vi "Insert_Event_Log(Auto_Event)vi.vi"(10 "[Log] 紀錄Auto流程":T1, 11 "DBlink":string="Driver={ODBC Driver 17 for SQL Server};Server=localhost\\SQLEXPRESS;Database=ZDX905;UID=labview;PWD=Dsa@54137926") -> (0 "error out":errorcluster, 3 "DBlink out":string)   [LabVIEW 2019]
uses:
  <vilib>/addons/database/Connection.llb/DB Tools Open Connec (String).vi
  <vilib>/addons/database/NI_Database_API.lvlib
panel:
  in  "error in (no error)":errorcluster
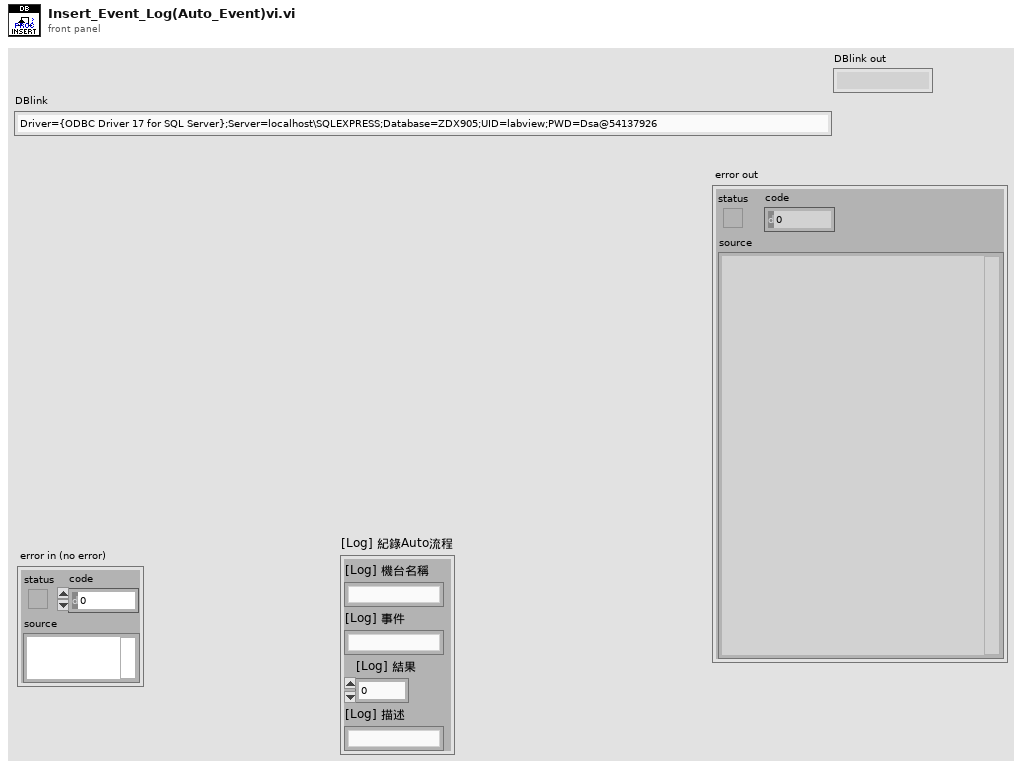
[diagram p1: front panel]
types:
  T1 = cluster{"[Log] 機台名稱":string, "[Log] 事件":string, "[Log] 結果":u16, "[Log] 描述":string}
  T2 = typedef "NI_Database_API.lvlib/Conn ObjectReference.ctl" = refnum<k1>
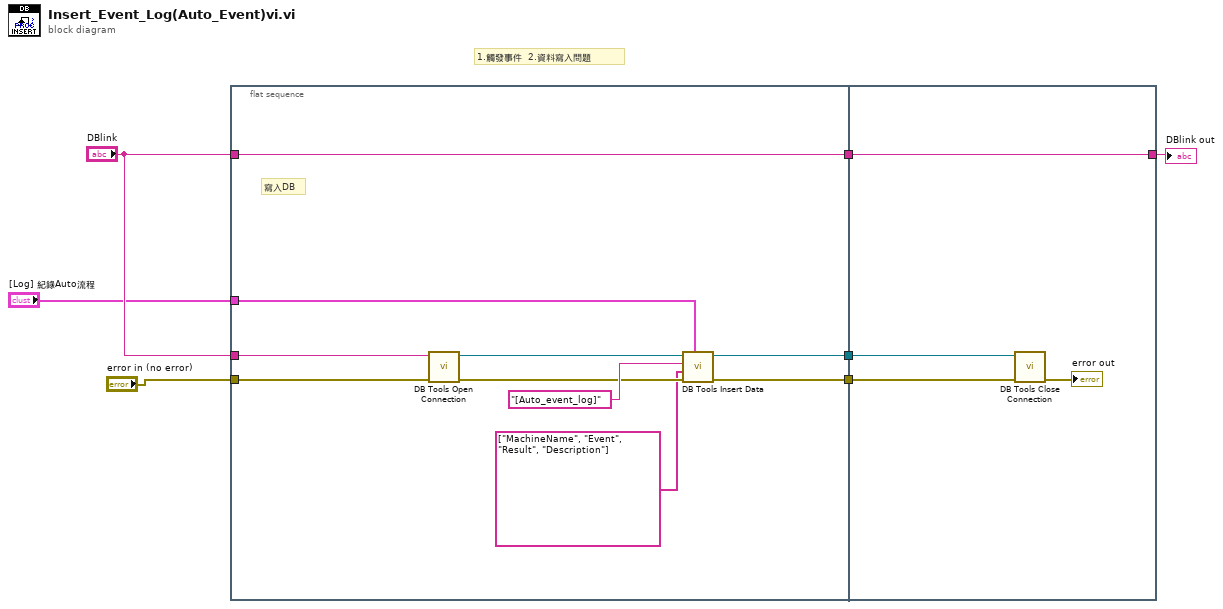
[diagram p0: block diagram]
diagram:
  # "1.觸發事件  2.資料寫入問題"
  n1 = flat-sequence {
    tunnel: [w16] -> w7
    tunnel: [w17] -> w6
    tunnel: "error in (no error)" -> [w11]
    tunnel: "DBlink" -> [w10]
    tunnel: "DBlink" -> [w9]
    tunnel: [w9] -> w3
    tunnel: "[Log] 紀錄Auto流程" -> [w8]
    tunnel: w7 -> [w19]
    tunnel: w6 -> [w20]
    tunnel: w3 -> [w18]
    tunnel: [w18] -> w2
    frame #0 {
      # "寫入DB"
      n2 = call-poly <vilib>:"DB Tools Open Connection.vi"("error in (no error)"=w11, "connection information"=w10) -> ("error out"=w14:errorcluster, "connection reference"=w13:T2)  [unwired: 6 in]
      n3 = call <vilib>:"DB Tools Insert Data.vi"("data"=w8, "error in (no error)"=w14, "columns"=string[] ["MachineName", "Event", "Result", "Description"], "table"="[Auto_event_log]", "connection reference"=w13) -> ("error out"=w16:errorcluster, "connection reference out"=w17:T2)  [unwired: 5 in]
    }
    frame #1 {
      n4 = call <vilib>:"DB Tools Close Connection.vi"("error in (no error)"=w19, "connection reference"=w20) -> ("error out"=→"error out":errorcluster)  [unwired: 5 in]
    }
  }
  "DBlink out" <- w2
